vi "CMD_SERIALCLOSE.vi"(6 "Gantry in":refnum<class "Gantry.lvclass">, 7 "Console Log in":refnum<class "Console Log.lvclass">, 8 "error in (no error)":errorcluster, 10 "Arguments":string[](array[string]), 11 "gScript Interpreter in":refnum<class "gScript Interpreter.lvclass">) -> (0 "error out":errorcluster, 3 "gScript Interpreter out":refnum<class "gScript Interpreter.lvclass">, 4 "Gantry out":refnum<class "Gantry.lvclass">, 5 "Console Log out":refnum<class "Console Log.lvclass">)   [LabVIEW 2024, in "gScript Interpreter.lvclass"]
uses:
  gScript Interpreter.lvclass
  Shared Components/Gantry Class/Gantry.lvclass
  Application Utilities/Console Log/Console Log.lvclass
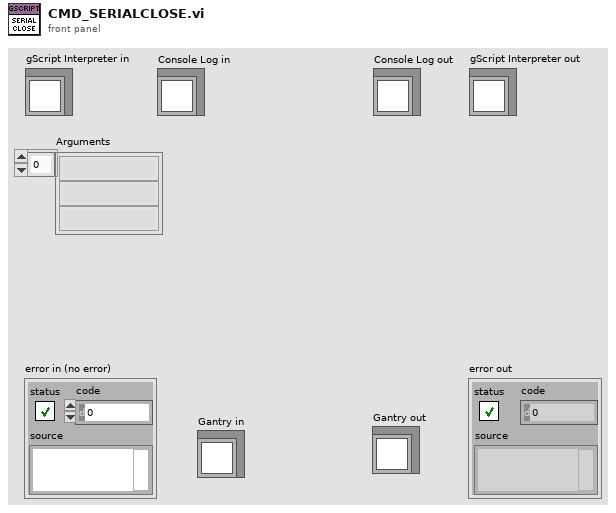
[diagram p1: front panel]
types:
  T1 = typedef "Memory Cell.ctl" = cluster{"type":T2, "x":dbl, "y":dbl, "z":dbl, "w":dbl}
  T2 = typedef "Memory Cell Type Enum.ctl" = enum16{"integer", "float", "vector", "rotation"}
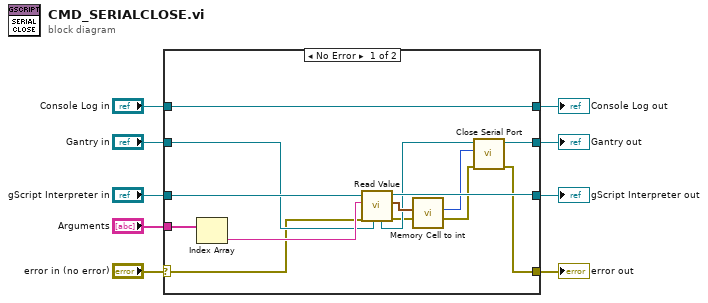
[diagram p0: block diagram]
diagram:
  n1 = case shown="No Error" "error in (no error)" {
    selector: "error in (no error)" -> [w15 w26]
    tunnel: [w10 w26] -> w8
    tunnel: [w18 w25] -> w6
    tunnel: "gScript Interpreter in" -> [w17 w25]
    tunnel: "Arguments" -> [w21 _]
    tunnel: "Gantry in" -> [w16 w24]
    tunnel: [w13 w24] -> w3
    tunnel: "Console Log in" -> [w22 w23]
    tunnel: [w22 w23] -> w1
    frame No Error {
      n2 = Index Array(array=w21) -> (element=w20:string)  [unwired: 1 in]
      n3 = call-dynamic "Read Value.vi"("Gantry in"=w16, "error in (no error)"=w15, "String in"=w20, "gScript Interpreter in"=w17) -> ("error out"=w11:errorcluster, "Memory Cell"=w19:T1, "gScript Interpreter out"=w18:refnum<class "gScript Interpreter.lvclass">, "Gantry out"=w14:refnum<class "Gantry.lvclass">)  [unwired: 4 in]
      n4 = call "Memory Cell to int.vi"("Memory Cell"=w19) -> ("Int out"=w12:i32)  [unwired: 10 in]
      n5 = call "Close Serial Port.vi"("error in (no error)"=w11, "Connection ID"=w12, "Gantry in"=w14) -> ("error out"=w10:errorcluster, "Gantry out"=w13:refnum<class "Gantry.lvclass">)  [unwired: 7 in]
    }
    frame Error {
    }
  }
  "error out" <- w8
  "gScript Interpreter out" <- w6
  "Gantry out" <- w3
  "Console Log out" <- w1
